vi "_UploadFirmware.vi"() -> ()   [LabVIEW 2016]
panel:
  out "name":string
  in  "Connect REPL":bool
  in  "Test":bool
  in  "Stop":bool
  in  "Connect":bool
  in  "VISA Refnum in":refnum<visa-resource-name>="ASRL32::INSTR"
  in  "Stage 2":bool
  in  "Stage 1":bool
  in  "Copy":bool
  out "PC files":string[](array[string])=["fwupdate.mpy", "PYBD_SF2_W4F2.dfu.gz", "PYBD_SF2_W4F2_mboot.dfu.gz"]
  out "Console":string="\r\n>>> \r\nPYB: sync filesystems\r\nPYB: soft reboot\r\nMicroPython v1.10-210-g45076ee50-dirty on 2019-02-02; PYBD_SF2 with STM32F722IEK\r\nType \"help()\" for more information.\r\n>>> \r\n>>> import fwupdate\r\n>>> fwupdate.stage1()\r\nLoading file /flash/PYBD_SF2_W4F2_mboot.dfu.gz\r\nSupplied version of mboot is already on device.\r\nstage1 done, rebooting\r\nMicroPython v1.10-210-g45076ee50-dirty on 2019-02-02; PYBD_SF2 with STM32F722IEK\r\nType \"help()\" for more information.\r\n>>> \r\n>>> import fwupdate\r\n>>> fwupdate.stage2()\r\nstage2 done\r\n>>> \r\nPYB: sync filesystems\r\nPYB: soft reboot\r\nMicroPython v1.10-210-g45076ee50-dirty on 2019-02-02; PYBD_SF2 with STM32F722IEK\r\nType \"help()\" for more information.\r\n>>> \r\n>>> "
  # "1. Select your serial port\n2. connect up\n3. copy over the files to the Pyboard - and wait for them  \n          to copy over (it takes 30 sec)\n4. flash stage 1 - and wait for the lights to stop blinking (\n          it takes 30 sec)\n5. flash stage 2 and run a test"
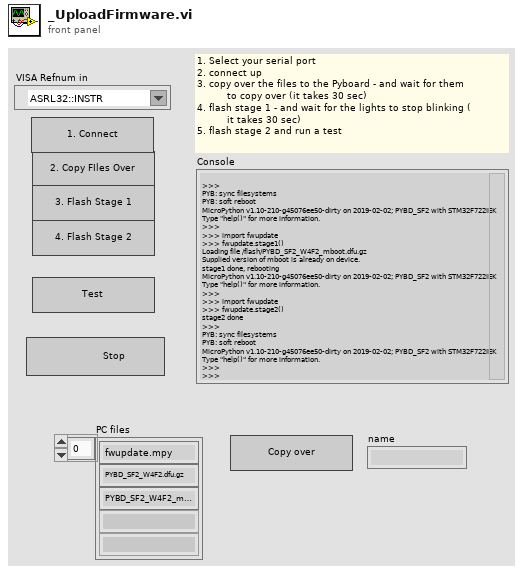
[diagram p1: front panel]
types:
  T1 = enum8{"Enabled", "Disabled", "Disabled and Grayed Out"}
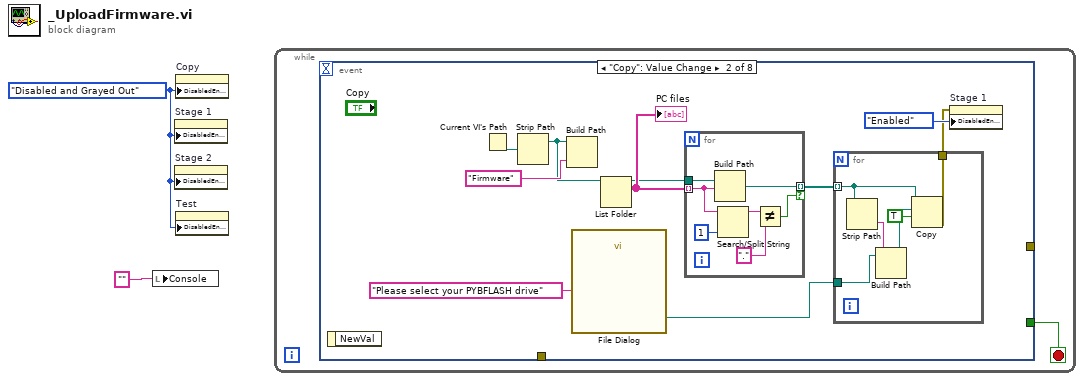
[diagram p0: block diagram]
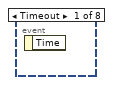
[diagram p2: hidden frame]
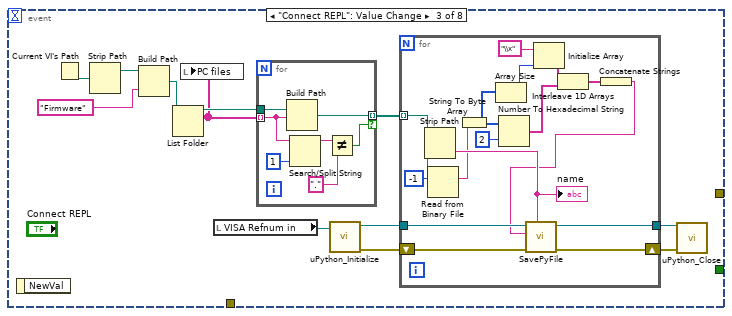
[diagram p3: hidden frame]
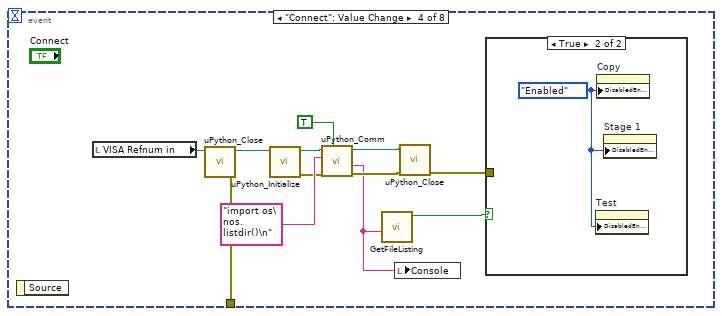
[diagram p4: hidden frame]
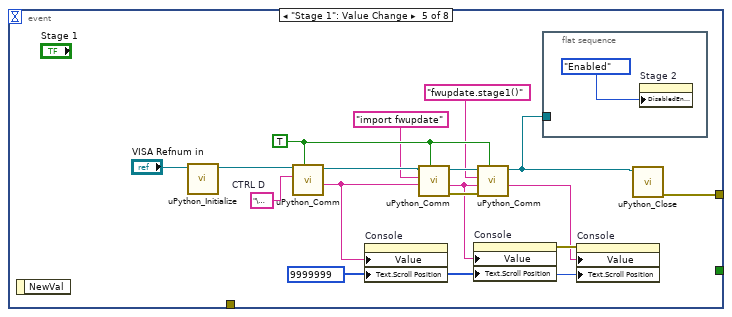
[diagram p6: hidden frame]
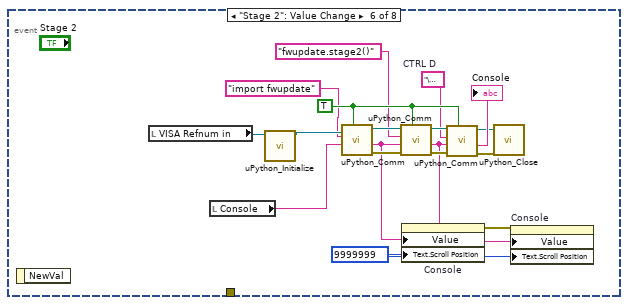
[diagram p7: hidden frame]
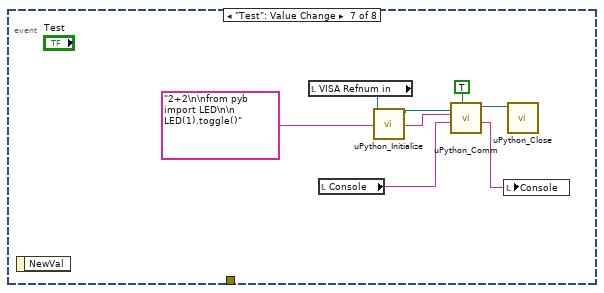
[diagram p8: hidden frame]
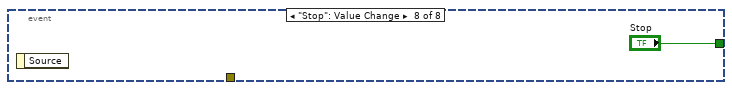
[diagram p9: hidden frame]
diagram:
  w2 = T1."Disabled and Grayed Out" ("Disabled")
  n1 = local write "Console"("") -> ()
  n2 = property on="Stage 1" class="Bool"("DisabledEnum"=w2) -> ()  [unwired: 2 in, 2 out]
  n3 = property on="Stage 2" class="Bool"("DisabledEnum"=w2) -> ()  [unwired: 2 in, 2 out]
  n4 = property on="Copy" class="Bool"("DisabledEnum"=w2) -> ()  [unwired: 2 in, 2 out]
  n5 = property on="Test" class="Bool"("DisabledEnum"=w2) -> ()  [unwired: 2 in, 2 out]
  n6 = while {
    stop <- w3 stop-if-true
    n7 = event shown="[1] \"Copy\": Value Change" {
      selector: _ -> [_ _ _ _ _ _ _ _]
      dyn-events: _ -> [_ _ _ _ _ _ _ _]
      timeout: _ -> [_ _ _ _ _ _ _ _]
      tunnel: [_ _ _ _ _ _ _ "Stop"] -> w3
      tunnel: [_ _ _ _ w81 _ _ _] -> _
      tunnel: [_ _ _ w62 _ _ _ _] -> _
      event Timeout {
        n8 = event-data() -> ()  [unwired: 1 in, 1 out]
      }
      event "Copy": Value Change {
        n9 = event-data() -> ()  [unwired: 1 in, 1 out]
        n10 = Current VI's Path() -> (path=w9:path)
        n11 = Strip Path(path=w9) -> (stripped path=w4:path)  [unwired: 1 out]
        n12 = Build Path(base path=w4, name or relative path="Firmware") -> ()  [unwired: 1 out]
        n13 = call "File Dialog"("prompt"="Please select your PYBFLASH drive") -> ("selected path"=w13:path)  [unwired: 11 in, 3 out]
        n14 = List Folder(path=w4) -> (path out=w10:path, filenames=w11:string[])  [unwired: 3 in, 2 out]
        "PC files" <- w11
        n15 = for {
          tunnel: w10 -> [w26]
          tunnel: w11 -> [w24] mode=indexing
          tunnel: [w25] -> w12 mode=indexing if=w20
          n16 = Build Path(base path=w26, name or relative path=w24) -> (appended path=w25:path)
          n17 = Search/Split String(string=w24, offset (0)=1) -> (substring before match=w22:string)  [unwired: 1 in, 2 out]
          n18 = Not Equal?(x=w22, y=".") -> (x != y?=w20:bool)
        }
        n19 = for {
          tunnel: w12 -> [w19] mode=indexing
          tunnel: w13 -> [w18]
          tunnel: [w14] -> w5
          n20 = Strip Path(path=w19) -> (name=w17:string)  [unwired: 1 out]
          n21 = Build Path(base path=w18, name or relative path=w17) -> (appended path=w16:path)
          n22 = Copy(9:TRUE ("overwrite (F)"), 10:w16, 11:w19) -> (0:w14:errorcluster)  [unwired: 2 in, 2 out]
        }
        n23 = property on="Stage 1" class="Bool"(error in=w5, "DisabledEnum"=T1."Enabled" ("Disabled")) -> ()  [unwired: 1 in, 2 out]
      }
      event "Connect REPL": Value Change {
        n24 = event-data() -> ()  [unwired: 1 in, 1 out]
        n25 = Current VI's Path() -> (path=w34:path)
        n26 = Strip Path(path=w34) -> (stripped path=w35:path)  [unwired: 1 out]
        n27 = Build Path(base path=w35, name or relative path="Firmware") -> (appended path=w37:path)
        n28 = List Folder(path=w37) -> (path out=w36:path, filenames=w32:string[])  [unwired: 3 in, 2 out]
        n29 = local write "PC files"(w32) -> ()
        n30 = local read "VISA Refnum in"() -> (w31:refnum<visa-resource-name>)
        n31 = for {
          tunnel: w36 -> [w61]
          tunnel: w32 -> [w59] mode=indexing
          tunnel: [w60] -> w38 mode=indexing if=w55
          n32 = Build Path(base path=w61, name or relative path=w59) -> (appended path=w60:path)
          n33 = Search/Split String(string=w59, offset (0)=1) -> (substring before match=w57:string)  [unwired: 1 in, 2 out]
          n34 = Not Equal?(x=w57, y=".") -> (x != y?=w55:bool)
        }
        n35 = call "uPython_Initialize.vi"("VISA Refnum in"=w31) -> ("error out"=w29:errorcluster, "VISA Refnum out"=w30:refnum<visa-resource-name>)  [unwired: 9 in]
        n36 = for {
          tunnel: w38 -> [w49] mode=indexing
          tunnel: w30 -> [w54]
          shift-right: [w52] -> w28
          shift-left: w29 -> [w53]
          tunnel: [w51] -> w27
          n37 = Strip Path(path=w49) -> (name=w50:string)  [unwired: 1 out]
          "name" <- w50
          n38 = Read from Binary File(10:-1 ("count (1)"), 11:w49) -> (2:w40:string)  [unwired: 4 in, 3 out]
          n39 = String To Byte Array(string=w40) -> (unsigned byte array=w44:u8[])
          n40 = Array Size(array=w44) -> (size(s)=w43:i32)
          n41 = Number To Hexadecimal String(1:i16 2 ("width (-)"), 2:w44) -> (0:w46:string[])
          n42 = Initialize Array("\\x" ("format string"), w43) -> (w42:string[])
          n43 = Interleave 1D Arrays(w42, w46) -> (w41:string[])
          n44 = Concatenate Strings(w41) -> (w39:string)
          n45 = call "SavePyFile.vi"("Name"=w50, "error in"=w53, "Python Code"=w39, "VISA in"=w54) -> ("error out"=w52:errorcluster, "VISA out"=w51:refnum<visa-resource-name>)  [unwired: 5 in, 1 out]
        }
        n46 = call "uPython_Close.vi"("error in"=w28, "VISA  in"=w27) -> ()  [unwired: 8 in, 2 out]
      }
      event "Connect": Value Change {
        n47 = event-data() -> ()  [unwired: 1 in, 1 out]
        n48 = local read "VISA Refnum in"() -> (w72:refnum<visa-resource-name>)
        n49 = call "uPython_Close.vi"("VISA  in"=w72) -> ("error out"=w62:errorcluster, "VISA  out"=w73:refnum<visa-resource-name>)  [unwired: 9 in]
        n50 = call "uPython_Initialize.vi"("VISA Refnum in"=w73) -> ("error out"=w66:errorcluster, "VISA Refnum out"=w71:refnum<visa-resource-name>)  [unwired: 9 in]
        n51 = call "uPython_Comm.vi"("Wait for Reply?"=TRUE, "error in (no error)"=w66, "Script"="import os\nos.listdir()\n", "VISA Refnum in"=w71) -> ("error out"=w65:errorcluster, "Console Out"=w63:string, "VISA out"=w68:refnum<visa-resource-name>)  [unwired: 3 in, 2 out]
        n52 = call "GetFileListing.vi"("Console In"=w63) -> ("Success?"=w67:bool)  [unwired: 9 in, 1 out]
        n53 = local write "Console"(w63) -> ()
        n54 = call "uPython_Close.vi"("error in"=w65, "VISA  in"=w68) -> ("error out"=w64:errorcluster)  [unwired: 8 in, 1 out]
        n55 = case shown="True" w67 {
          tunnel: w64 -> [_ _]
          frame False {
          }
          frame True {
            w74 = T1."Enabled" ("Disabled")
            n56 = property on="Test" class="Bool"("DisabledEnum"=w74) -> ()  [unwired: 2 in, 2 out]
            n57 = property on="Copy" class="Bool"("DisabledEnum"=w74) -> ()  [unwired: 2 in, 2 out]
            n58 = property on="Stage 1" class="Bool"("DisabledEnum"=w74) -> ()  [unwired: 2 in, 2 out]
          }
        }
      }
      event "Stage 1": Value Change {
        w77 = u32 9999999 ("Text.Selection:End")
        w85 = TRUE ("Wait for Reply?")
        w82 = "\u0004"  # CTRL D
        n59 = event-data() -> ()  [unwired: 1 in, 1 out]
        n60 = call "uPython_Initialize.vi"("VISA Refnum in"="VISA Refnum in") -> ("VISA Refnum out"=w86:refnum<visa-resource-name>)  [unwired: 9 in, 1 out]
        n61 = call "uPython_Comm.vi"("Wait for Reply?"=w85, "Script"=w82, "VISA Refnum in"=w86) -> ("Console Out"=w79:string, "VISA out"=w87:refnum<visa-resource-name>)  [unwired: 4 in, 3 out]
        n62 = property on="Console" class="Str"("Value"=w79, "Text.Scroll Position"=w77) -> ()  [unwired: 2 in, 2 out]
        n63 = call "uPython_Comm.vi"("Wait for Reply?"=w85, "Console In"=w79, "Script"="import fwupdate", "VISA Refnum in"=w87) -> ("error out"=w88:errorcluster, "Console Out"=w76:string, "VISA out"=w89:refnum<visa-resource-name>)  [unwired: 3 in, 2 out]
        n64 = property on="Console" class="Str"("Value"=w76, "Text.Scroll Position"=w77) -> (error out=w78:errorcluster)  [unwired: 2 in, 1 out]
        n65 = call "uPython_Comm.vi"("Wait for Reply?"=w85, "error in (no error)"=w88, "Console In"=w76, "Script"="fwupdate.stage1()", "VISA Refnum in"=w89) -> ("Console Out"=w75:string, "VISA out"=w80:refnum<visa-resource-name>)  [unwired: 2 in, 3 out]
        n66 = flat-sequence {
          tunnel: w80 -> [_]
          frame #0 {
            n67 = property on="Stage 2" class="Bool"("DisabledEnum"=T1."Enabled" ("Disabled")) -> ()  [unwired: 2 in, 2 out]
          }
        }
        n68 = property on="Console" class="Str"(error in=w78, "Value"=w75, "Text.Scroll Position"=w77) -> ()  [unwired: 1 in, 2 out]
        n69 = call "uPython_Close.vi"("VISA  in"=w80) -> ("error out"=w81:errorcluster)  [unwired: 9 in, 1 out]
      }
      event "Stage 2": Value Change {
        w94 = u32 9999999 ("Text.Selection:End")
        w102 = TRUE ("Wait for Reply?")
        w101 = "\u0004"  # CTRL D
        n70 = event-data() -> ()  [unwired: 1 in, 1 out]
        n71 = local read "VISA Refnum in"() -> (w96:refnum<visa-resource-name>)
        n72 = local read "Console"() -> (w98:string)
        n73 = call "uPython_Initialize.vi"("VISA Refnum in"=w96) -> ("VISA Refnum out"=w105:refnum<visa-resource-name>)  [unwired: 9 in, 1 out]
        n74 = call "uPython_Comm.vi"("Wait for Reply?"=w102, "Console In"=w98, "Script"="import fwupdate", "VISA Refnum in"=w105) -> ("error out"=w104:errorcluster, "Console Out"=w92:string, "VISA out"=w103:refnum<visa-resource-name>)  [unwired: 3 in, 2 out]
        n75 = call "uPython_Comm.vi"("Wait for Reply?"=w102, "error in (no error)"=w104, "Console In"=w92, "Script"="fwupdate.stage2()", "VISA Refnum in"=w103) -> ("error out"=w97:errorcluster, "Console Out"=w93:string, "VISA out"=w106:refnum<visa-resource-name>)  [unwired: 2 in, 2 out]
        n76 = property on="Console" class="Str"("Value"=w92, "Text.Scroll Position"=w94) -> (error out=w95:errorcluster)  [unwired: 2 in, 1 out]
        n77 = call "uPython_Comm.vi"("Wait for Reply?"=w102, "error in (no error)"=w97, "Console In"=w93, "Script"=w101, "VISA Refnum in"=w106) -> ("error out"=w107:errorcluster, "Console Out"=→"Console":string, "VISA out"=w108:refnum<visa-resource-name>)  [unwired: 2 in, 2 out]
        n78 = call "uPython_Close.vi"("error in"=w107, "VISA  in"=w108) -> ()  [unwired: 8 in, 2 out]
        n79 = property on="Console" class="Str"(error in=w95, "Value"=w93, "Text.Scroll Position"=w94) -> ()  [unwired: 1 in, 2 out]
      }
      event "Test": Value Change {
        n80 = event-data() -> ()  [unwired: 1 in, 1 out]
        n81 = local read "VISA Refnum in"() -> (w112:refnum<visa-resource-name>)
        n82 = local read "Console"() -> (w114:string)
        n83 = call "uPython_Initialize.vi"("VISA Refnum in"=w112) -> ("VISA Refnum out"=w116:refnum<visa-resource-name>)  [unwired: 9 in, 1 out]
        n84 = call "uPython_Comm.vi"("Wait for Reply?"=TRUE, "Console In"=w114, "Script"="2+2\n\nfrom pyb import LED\n\n     LED(1).toggle()", "VISA Refnum in"=w116) -> ("Console Out"=w113:string, "VISA out"=w110:refnum<visa-resource-name>)  [unwired: 3 in, 3 out]
        n85 = local write "Console"(w113) -> ()
        n86 = call "uPython_Close.vi"("VISA  in"=w110) -> ()  [unwired: 9 in, 2 out]
      }
      event "Stop": Value Change {
        n87 = event-data() -> ()  [unwired: 1 in, 1 out]
      }
    }
  }
